vi "Dut Rx Abort.vi"(0 "MTK7615 in":refnum<class "MTK7615.lvclass">, 11 "error in (no error)":errorcluster) -> (4 "MTK7615 out":refnum<class "MTK7615.lvclass">, 15 "error out":errorcluster)   [LabVIEW 2015, in "MTK7615.lvlib" / "MTK7615.lvclass"]
uses:
  MTK7615.lvclass
  MTK7615.lvclass/MTK7615.ctl
panel:
  out "Packets":i32
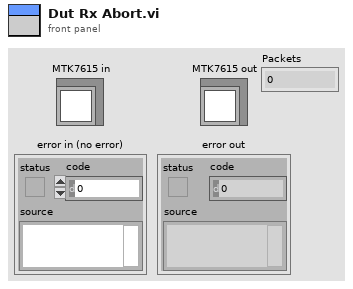
[diagram p1: front panel]
types:
  T1 = typedef "niDCT_TELNET_PrivRef.ctl" = refnum<data-value>
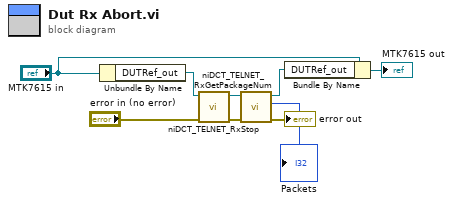
[diagram p0: block diagram]
diagram:
  n1 = Unbundle By Name("MTK7615 in") -> ("DUTRef_out"=w9:T1)
  n2 = call "niDCT_TELNET_RxStop.vi"("error in (no error)"="error in (no error)", "DUTRef"=w9) -> ("error out"=w4:errorcluster, "DUTRef_out"=w5:T1)  [unwired: 8 in]
  n3 = call "niDCT_TELNET_RxGetPackageNum.vi"("error in (no error)"=w4, "DUTRef"=w5) -> ("error out"=→"error out":errorcluster, "Packets"=→"Packets":i32, "DUTRef_out"=w2:T1)  [unwired: 7 in]
  n4 = Bundle By Name(cluster="MTK7615 in", "DUTRef_out"=w2) -> (→"MTK7615 out":refnum<class "MTK7615.lvclass">)
